vi "故障码字段定义.vi"(11 "故障代码":u16) -> (3 "字符串":string)   [LabVIEW 2016, in "斯坦道氨氮.lvlib"]
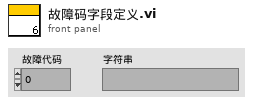
[diagram p1: front panel]
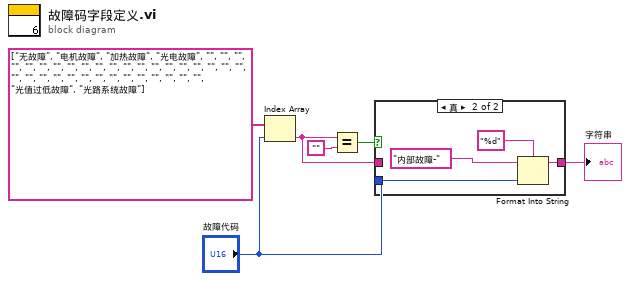
[diagram p0: block diagram]
diagram:
  n1 = Index Array(array=string[] ["无故障", "电机故障", "加热故障", "光电故障", "", "", "", "", "", "", "", "", "", "", "", "", "", "", "", "", "", "", "", "", "", "", "", "", "", "", "", "", "", "", "", "", "", "", "光值过低故障", "光路系统故障"], index="故障代码") -> (element=w4:string)
  n2 = Equal?(x=w4, y="") -> (x = y?=w5:bool)
  n3 = case shown="真" w5 {
    tunnel: [w7 w9] -> w3
    tunnel: w4 -> [w7 _]
    tunnel: "故障代码" -> [_ w8]
    frame False {
    }
    frame True {
      n4 = Format Into String(format string="%d" ("格式字符串"), initial string="内部故障-" ("工作状态"), w8) -> (resulting string=w9:string)  [unwired: 1 in, 1 out]
    }
  }
  "字符串" <- w3
